vi "Climb Speed Logic Sub.vi"(6 "Climb Speed":dbl=-55.0, 8 "Hump Speed":dbl=-70.0, 9 "y":dbl, 10 "Arm Current":dbl, 11 "Numeric":dbl) -> (3 "f":dbl)   [LabVIEW 2012]
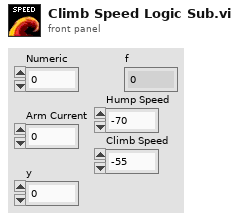
[diagram p1: front panel]
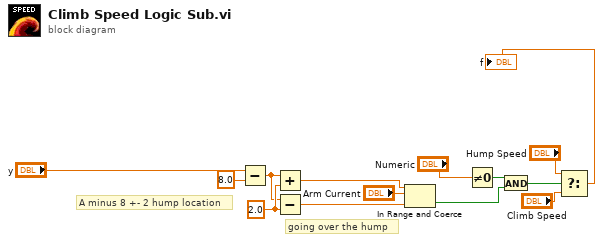
[diagram p0: block diagram]
diagram:
  w11 = 2.0 ("y")
  # "A minus 8 +- 2 hump location"
  # "going over the hump"
  n1 = Subtract(x="y", y=8.0) -> (x-y=w10:dbl)
  n2 = Add(x=w10, y=w11) -> (x+y=w6:dbl)
  n3 = Subtract(x=w10, y=w11) -> (x-y=w7:dbl)
  n4 = In Range and Coerce(upper limit=w6, x="Arm Current", lower limit=w7) -> (In Range?=w5:bool)  [unwired: 1 out]
  n5 = Not Equal To 0?(x="Numeric") -> (x != 0?=w12:bool)
  n6 = And(x=w12, y=w5) -> (x .and. y?=w4:bool)
  n7 = Select(t="Hump Speed", s=w4, f="Climb Speed") -> (s? t:f=→"f":dbl)
